vi "load_cell_read_subvi.vi"(11 "Bytes Read":u8[](array[numeric])) -> (3 "Numeric":u32)   [LabVIEW 2021]
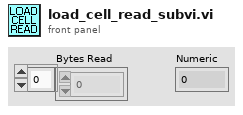
[diagram p1: front panel]
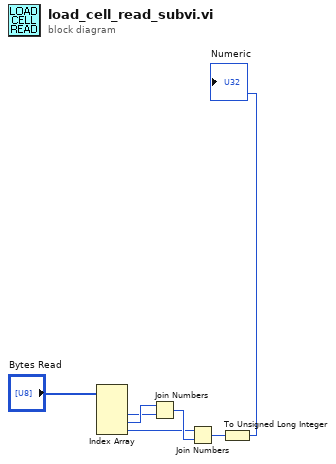
[diagram p0: block diagram]
diagram:
  n1 = Index Array(array="Bytes Read") -> (element #2=w2:u8, element #3=w3:u8, element #4=w4:u8)  [unwired: 4 in, 1 out]
  n2 = Join Numbers(hi=w3, lo=w2) -> ((hi.lo)=w5:u16)
  n3 = Join Numbers(hi=w4, lo=w5) -> ((hi.lo)=w1:u32)
  n4 = To Unsigned Long Integer(number=w1) -> (unsigned 32bit integer=→"Numeric":u32)
